vi "Locate Error Tunnels on Case.vi"(8 "error in (no error)":errorcluster, 11 "CaseSel Refnum In":refnum<vi>) -> (0 "error out":errorcluster, 1 "Error In Tunnel":refnum<vi>, 2 "Error Out Tunnel":refnum<vi>, 3 "CaseSel Refnum":refnum<vi>)   [LabVIEW 2018]
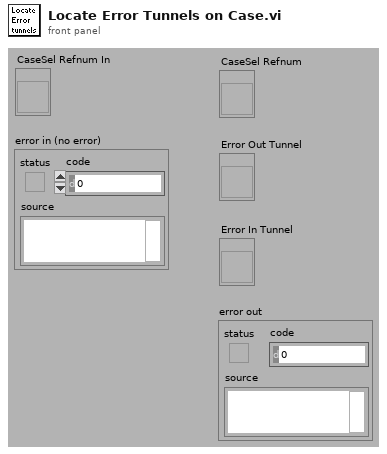
[diagram p1: front panel]
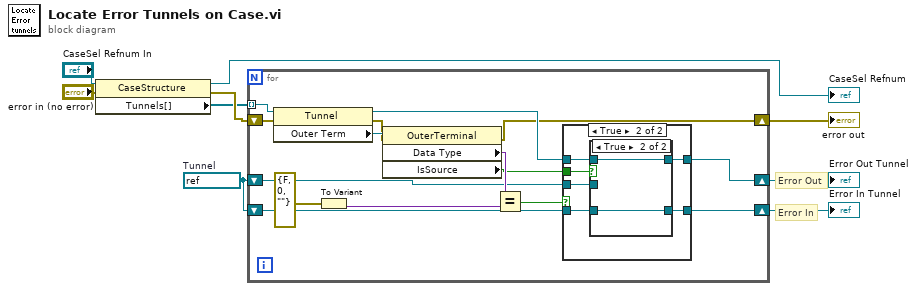
[diagram p0: block diagram]
diagram:
  w5 = refnum<vi> refnum  # Tunnel
  # "Error In"
  # "Error Out"
  n1 = property class="CaseStructure"(reference="CaseSel Refnum In", error in="error in (no error)") -> (reference out=→"CaseSel Refnum":refnum<vi>, error out=w4:errorcluster, "Tunnels[]"=w3:refnum<vi>[])
  n2 = for {
    tunnel: w3 -> [w23] mode=indexing
    shift-right: [w10] -> w6
    shift-left: w4 -> [w24]
    shift-right: [w14] -> w8
    shift-left: w5 -> [w12]
    shift-right: [w13] -> w9
    shift-left: w5 -> [w11]
    n3 = property class="Tunnel"(reference=w23, error in=w24) -> (reference out=w15:refnum<vi>, error out=w21:errorcluster, "Outer Term"=w22:refnum<vi>)
    n4 = To Variant(anything=errorcluster {"status"=FALSE, "code"=0, "source"=""} ("error out")) -> (Variant=w18:variant)
    n5 = property class="OuterTerminal"(reference=w22, error in=w21) -> (error out=w10:errorcluster, "Data Type"=w19:variant, "IsSource"=w16:bool)  [unwired: 1 out]
    n6 = Equal?(x=w19, y=w18) -> (x = y?=w17:bool)
    n7 = case shown="True" w17 {
      tunnel: w16 -> [_ w32]
      tunnel: w15 -> [w26 w31]
      tunnel: [w26 w30] -> w14
      tunnel: [w25 w29] -> w13
      tunnel: w12 -> [_ w28]
      tunnel: w11 -> [w25 w27]
      frame False {
      }
      frame True {
        n8 = case shown="True" w32 {
          tunnel: w31 -> [w34 w36]
          tunnel: [w33 w36] -> w30
          tunnel: [w34 w35] -> w29
          tunnel: w28 -> [w33 _]
          tunnel: w27 -> [_ w35]
          frame False {
          }
          frame True {
          }
        }
      }
    }
  }
  "Error In Tunnel" <- w9
  "Error Out Tunnel" <- w8
  "error out" <- w6
